vi "Accept TLS.vi"(7 "timeout ms":i32, 8 "error in (no error)":errorcluster, 10 "immutable TLS configuration":refnum<k36>, 11 "TCP Stream in":refnum<class "TCP Stream.lvclass">) -> (0 "error out":errorcluster, 2 "client certificate chain":cluster{"certificate":u8[]}[](array[cluster]), 3 "TCP Stream out":refnum<class "TCP Stream.lvclass">)   [LabVIEW 2020, in "Stream-TCP.lvlib" / "TCP Stream.lvclass"]
uses:
  TCP Stream.lvclass
  TCP Stream.lvclass/TCP Stream.ctl
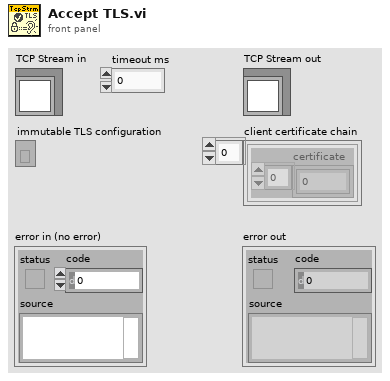
[diagram p1: front panel]
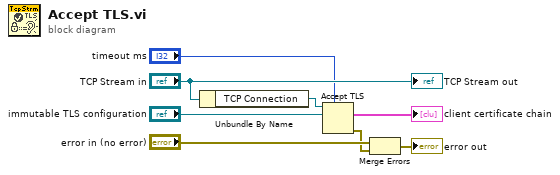
[diagram p0: block diagram]
diagram:
  n1 = Unbundle By Name("TCP Stream in") -> ("TCP Connection"=w6:refnum<k5>)
  n2 = Accept TLS(7:"timeout ms", 10:"immutable TLS configuration", 11:w6) -> (0:w3:errorcluster, 2:→"client certificate chain":cluster{"certificate":u8[]}[])  [unwired: 1 in, 1 out]
  n3 = Merge Errors("error in (no error)", w3) -> (→"error out":errorcluster)
  "TCP Stream out" <- "TCP Stream in"
